vi "Test_DIGIT_5122_Standalone_SubVIs.vi"(6 "Accum Number":i16, 7 "Use Software Trigger":bool=TRUE, 8 "error in (no error)":errorcluster, 9 "DATA Inputs":T3={"Record Length"=1000000, "Sample Rate"=10000000.0, "Data Type"=0, "Vertical Range"=10.0, "Acquisition Duration"=1.0} {"Vertical Range" items=["0.2"=0.2, "0.4"=0.4, "1"=1.0, "2"=2.0, "4"=4.0, "10"=10.0]; "Data Type" items=["I16", "DBL"]; "Sample Rate" items=["1 MHz"=1000000.0, "2 MHz"=2000000.0, "5 MHz"=5000000.0, "10 MHz"=10000000.0, "20 MHz"=20000000.0, "25 MHz"=25000000.0, "50 MHz"=50000000.0, "100 MHz"=100000000.0]}) -> (0 "error out":errorcluster)   [LabVIEW 2018]
doc: "This VI is a standalone test for the PXIe-5122 digitizer.\n\nIf software trigger is used, the acquisition starts immediately reading channel 0.\nIf an external trigger is used, please connect a TTL trigger to the EXT TRIG connector in front panel of the PXIe-5122 board."
uses:
  controls/DATA_Inputs.ctl
  controls/DIGIT_5122_Inputs.ctl
  <instrlib>/niScope/Controls/niScope trigger source.ctl
panel:
  out "Freq Spectrum":cluster{sgl[], sgl[]}(graph)
  in  "Number Of Acquisitions":i32
  in  "DIGIT 5122 Inputs":T1={"Sample Rate"=10000.0, "Resource Name"="DIGIT_5122", "Channel Name"="0", "Trigger Source"="VAL_EXTERNAL", "Vertical Range"=10.0, "Trigger Level"=3.0} {"Trigger Level" format="%.2f"; "Vertical Range" format="%.2f"; "Sample Rate" step=65535.0 format="%#_3p"}
  out "Graphe":i16[][](graph)
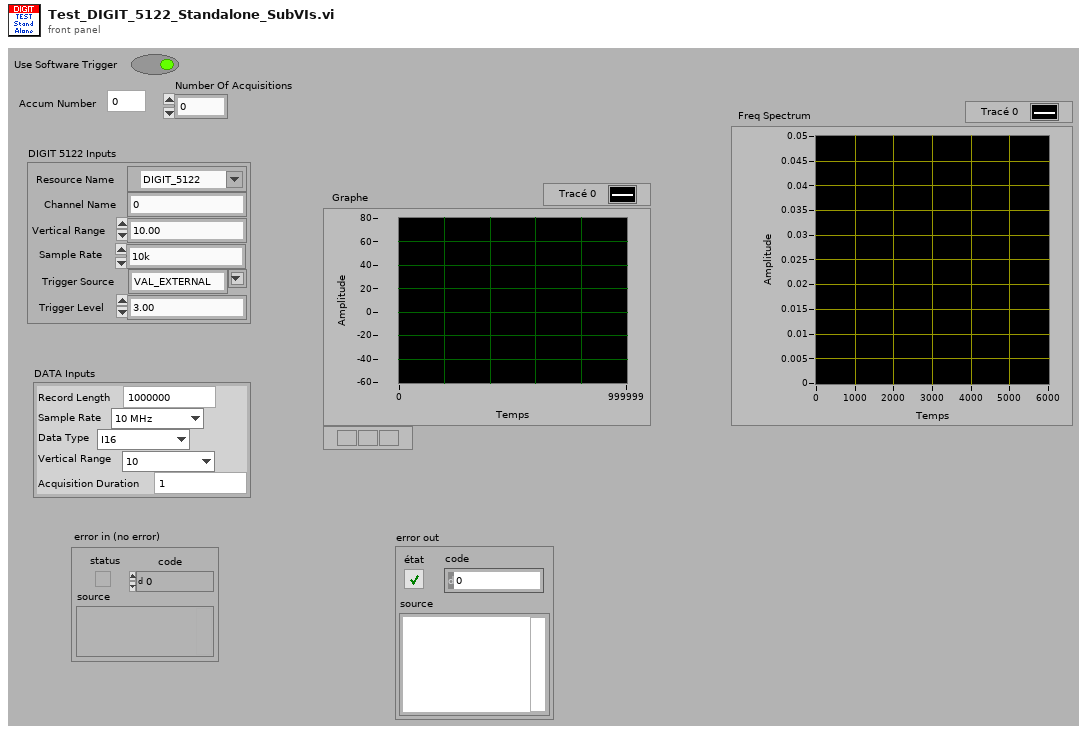
[diagram p1: front panel]
types:
  T1 = typedef "DIGIT_5122_Inputs.ctl" = cluster{"Sample Rate":dbl, "Resource Name":refnum<k15>, "Channel Name":string, "Trigger Source":T2, "Vertical Range":dbl, "Trigger Level":dbl}
  T2 = typedef "niScope trigger source.ctl" = string
  T3 = typedef "DATA_Inputs.ctl" = cluster{"Record Length":i32, "Sample Rate":dbl, "Data Type":u8, "Vertical Range":dbl, "Acquisition Duration":dbl}
  T4 = cluster{"actualSamples":i32, "absoluteInitialX":dbl, "relativeInitialX":dbl, "xIncrement":dbl, "offset":dbl, "gain":dbl, "reserved1":dbl, "reserved2":dbl}[]
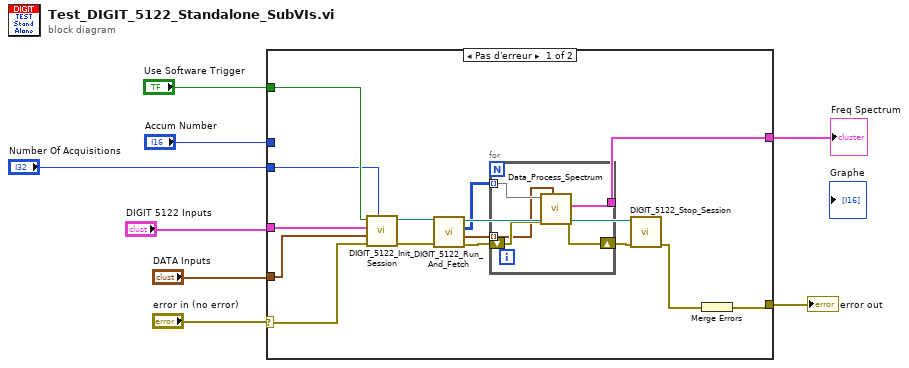
[diagram p0: block diagram]
diagram:
  n1 = case shown="Pas d'erreur" "error in (no error)" {
    selector: "error in (no error)" -> [w23 w29]
    tunnel: [w15 w29] -> w7
    tunnel: "Use Software Trigger" -> [w21 _]
    tunnel: "DIGIT 5122 Inputs" -> [w22 _]
    tunnel: "DATA Inputs" -> [w14 _]
    tunnel: "Accum Number" -> [_ _]
    tunnel: "Number Of Acquisitions" -> [w13 _]
    tunnel: [w12 _] -> w1
    frame No Error {
      n2 = call "DIGIT_5122_Init_Session.vi"("Number of Acquisitions"=w13, "error in (no error)"=w23, "DATA Inputs"=w14, "DIGIT 5122 Inputs"=w22, "Use Software Trigger"=w21) -> ("error out"=w20:errorcluster, "instrument handle out"=w19:refnum<k15>)  [unwired: 5 in]
      n3 = call "DIGIT_5122_Run_And_Fetch.vi"("error in (no error)"=w20, "instrument handle"=w19) -> ("error out"=w18:errorcluster, "wfm info"=w10:T4, "dataset"=w11:i16[][], "instrument handle out"=w17:refnum<k15>)  [unwired: 6 in]
      n4 = for {
        tunnel: [w26] -> w12
        tunnel: w11 -> [w25] mode=indexing
        tunnel: w10 -> [w24] mode=indexing
        shift-right: [w27] -> w9
        shift-left: w18 -> [w28]
        n5 = call "Data_Process_Spectrum.vi"("wfm info"=w24, "error in"=w28, "dataset"=w25) -> ("error out"=w27:errorcluster, "Frequency Spectrum"=w26:cluster{sgl[], sgl[]})  [unwired: 6 in, 1 out]
      }
      n6 = call "DIGIT_5122_Stop_Session.vi"("error in (no error)"=w9, "instrument handle"=w17) -> ("error out"=w16:errorcluster)  [unwired: 9 in]
      n7 = Merge Errors(w16) -> (w15:errorcluster)
    }
    frame Error {
    }
  }
  "error out" <- w7
  "Freq Spectrum" <- w1
